vi "MoveToStrip.vi"(6 "Single Needle":bool, 8 "Error In":errorcluster, 9 "Strip No.":u16, 10 "Region":u16, 11 "ProbeStationControl in":refnum<class "ProbeStationControl.lvclass">) -> (0 "Error Out":errorcluster, 2 "Z [µm]":i32, 3 "ProbeStationControl out":refnum<class "ProbeStationControl.lvclass">)   [LabVIEW 2018]
doc: "Move to specified strip index and touch down probe."
uses:
  InstrControl/ProbeStationControl/ProbeStationControl.lvclass
  InstrControl/ProbeStationControl/TeslaVelox/TeslaVeloxProbeStation.lvclass
  ProbePlanParams.vi
panel:
  out "Is Valid?":bool
  out "Axis":enum16{"X", "Y", "Z", "Theta"}(ring)
  out "Coordinate IN":i32
  out "Coordinate system":enum16{"Cartesian", "X as index"}(ring)
  out "previous Z [µm]":i32
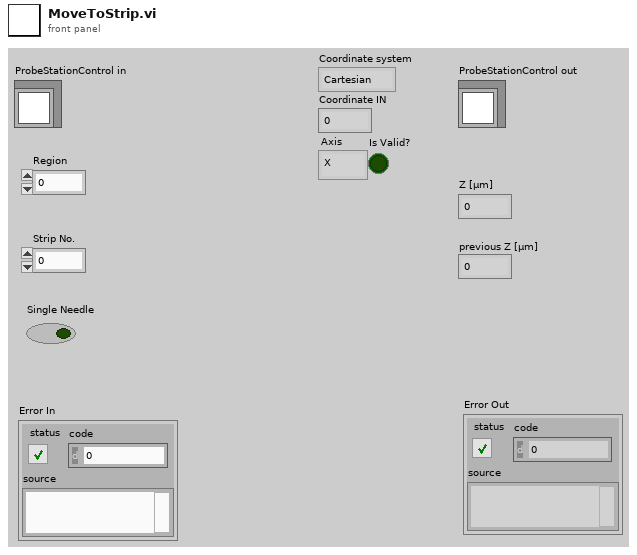
[diagram p1: front panel]
types:
  T1 = cluster{"Strip Number OUT":i32, "X0":i32, "Y0":i32, "X1":i32, "Y1":i32, "Xref":dbl, "Yref":dbl, "ProbePlan type":u32, "Inner pads offset":ext, "Outer pads offset":ext, "l_inner":ext, "l_outer":ext, "strip numbering":u16, "Device Orientation":ext, "Stagger offset":i32, "Yoffset":dbl, "Strip pitch":dbl, "Fiducail separation":dbl, "Radius":ext, "Relative strip angles":dbl, "Probeplan description":string, "ProbePlan array":cluster{"Region":string, "ProbePoints":cluster{"X":dbl, "Y":dbl, "Label":string, "CardViable?":bool}[]}[], "Test ProbePoints":cluster{"Regions Enabled":bool[], "From index":u32[], "To index":u32[]}}
  T2 = cluster{"Region":string, "ProbePoints":cluster{"X":dbl, "Y":dbl, "Label":string, "CardViable?":bool}[]}[]
  T3 = cluster{"Region":string, "ProbePoints":cluster{"X":dbl, "Y":dbl, "Label":string, "CardViable?":bool}[]}
  T4 = cluster{"X":dbl, "Y":dbl, "Label":string, "CardViable?":bool}[]
  T5 = cluster{"X":dbl, "Y":dbl, "Label":string, "CardViable?":bool}
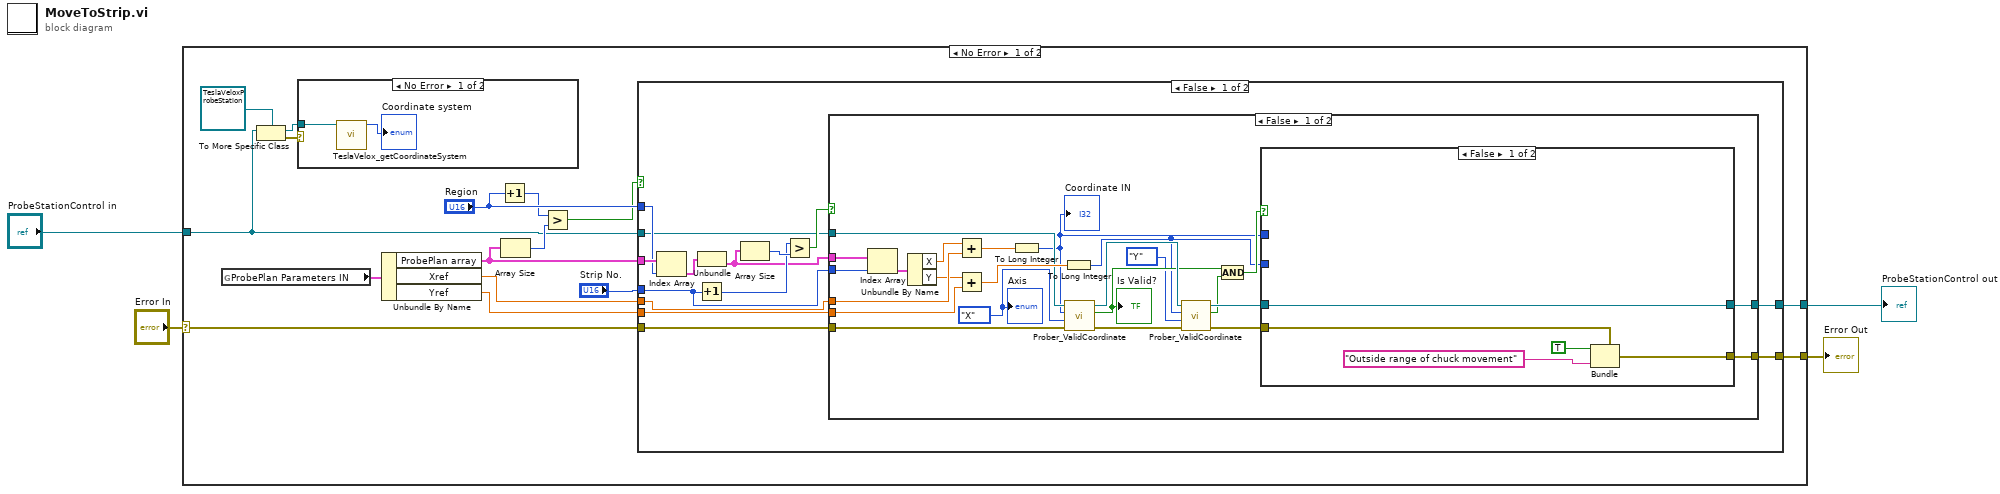
[diagram p0: block diagram]
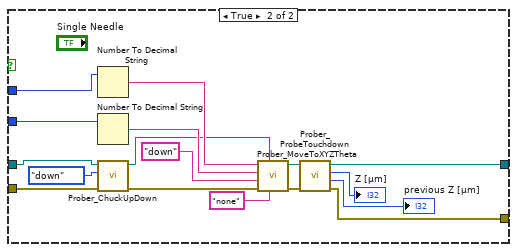
[diagram p3: hidden frame]
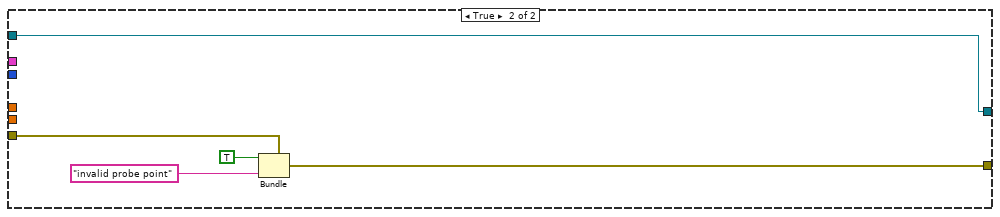
[diagram p4: hidden frame]
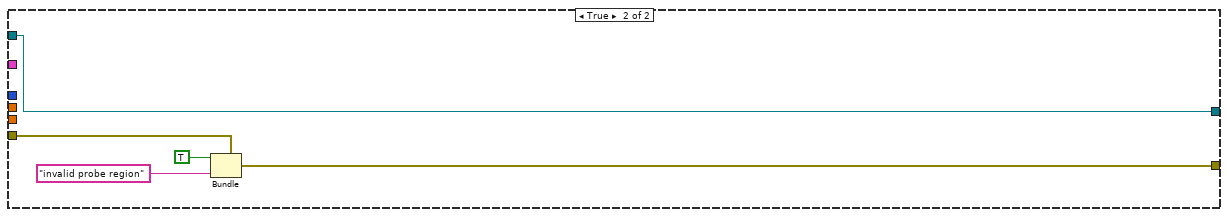
[diagram p5: hidden frame]
diagram:
  n1 = case shown="No Error" "Error In" {
    selector: "Error In" -> [w14 w93]
    tunnel: [w20 w93] -> w4
    tunnel: "ProbeStationControl in" -> [w8 w94]
    tunnel: [w9 w94] -> w1
    frame No Error {
      n2 = global read "ProbePlanParams.vi" "ProbePlan Parameters IN"() -> (w13:T1)
      n3 = To More Specific Class(target class=refnum<class "TeslaVeloxProbeStation.lvclass"> refnum ("TeslaVeloxProbeStation.lvclass"), reference=w8) -> (specific class reference=w7:refnum<class "TeslaVeloxProbeStation.lvclass">, error out=w5:errorcluster)  [unwired: 1 in]
      n4 = case shown="No Error" w5 {
        tunnel: w7 -> [w22 _]
        frame No Error {
          n5 = call "TeslaVelox_getCoordinateSystem.vi"("TeslaVeloxProbeStation.lvclass"=w22) -> ("Coordinate system"=→"Coordinate system":enum16{"Cartesian", "X as index"})  [unwired: 10 in]
        }
        frame Error {
        }
      }
      n6 = Unbundle By Name(w13) -> ("ProbePlan array"=w12:T2, "Xref"=w11:dbl, "Yref"=w10:dbl)
      n7 = Increment(x="Region") -> (x+1=w16:u16)
      n8 = Array Size(array=w12) -> (size(s)=w17:i32)
      n9 = Greater?(x=w16, y=w17) -> (0:w15:bool)
      n10 = case shown="False" w15 {
        tunnel: w14 -> [w31 w92]
        tunnel: [w30 w91] -> w20
        tunnel: "Region" -> [w34 _]
        tunnel: "Strip No." -> [w25 _]
        tunnel: w12 -> [w35 _]
        tunnel: w10 -> [w28 _]
        tunnel: w11 -> [w27 _]
        tunnel: [w24 w88] -> w9
        tunnel: w8 -> [w23 w88]
        frame False {
          n11 = Index Array(array=w35, index=w34) -> (element=w36:T3)
          n12 = Increment(x=w25) -> (x+1=w32:u16)
          n13 = Unbundle(w36) -> ("ProbePoints"=w26:T4)  [unwired: 1 out]
          n14 = Array Size(array=w26) -> (size(s)=w33:i32)
          n15 = Greater?(x=w32, y=w33) -> (0:w29:bool)
          n16 = case shown="False" w29 {
            tunnel: w31 -> [w48 w86]
            tunnel: [w53 w85] -> w30
            tunnel: w28 -> [w60 _]
            tunnel: w27 -> [w59 _]
            tunnel: w26 -> [w58 _]
            tunnel: w25 -> [w57 _]
            tunnel: [w50 w83] -> w24
            tunnel: w23 -> [w49 w83]
            frame False {
              w37 = enum16{"X", "Y", "Z", "Theta"}."X" ("Axis")
              n17 = Index Array(array=w58, index=w57) -> (element=w56:T5)
              n18 = Unbundle By Name(w56) -> ("X"=w55:dbl, "Y"=w54:dbl)
              n19 = Add(x=w55, y=w59) -> (x+y=w52:dbl)
              n20 = Add(x=w54, y=w60) -> (x+y=w51:dbl)
              n21 = To Long Integer(number=w52) -> (32bit integer=w38:i32)
              "Coordinate IN" <- w38
              n22 = To Long Integer(number=w51) -> (32bit integer=w40:i32)
              n23 = call-dynamic "Prober_ValidCoordinate.vi"("error in (no error)"=w48, "Axis"=w37, "Coordinate IN"=w38, "ProbeStationControl in"=w49) -> ("error out"=w47:errorcluster, "Is Valid?"=w42:bool, "ProbeStationControl out"=w45:refnum<class "ProbeStationControl.lvclass">)  [unwired: 5 in]
              "Is Valid?" <- w42
              n24 = call-dynamic "Prober_ValidCoordinate.vi"("error in (no error)"=w47, "Axis"=enum16{"X", "Y", "Z", "Theta"}."Y", "Coordinate IN"=w40, "ProbeStationControl in"=w45) -> ("error out"=w46:errorcluster, "Is Valid?"=w43:bool, "ProbeStationControl out"=w44:refnum<class "ProbeStationControl.lvclass">)  [unwired: 5 in]
              n25 = And(x=w42, y=w43) -> (x .and. y?=w41:bool)
              n26 = case shown="False" w41 {
                tunnel: w46 -> [w63 w66]
                tunnel: [w62 w77] -> w53
                tunnel: w38 -> [_ w82]
                tunnel: w40 -> [_ w81]
                tunnel: [w61 w76] -> w50
                tunnel: w44 -> [w61 w67]
                frame False {
                  n27 = Bundle(cluster=w63, "status"=TRUE, "source"="Outside range of chuck movement") -> (w62:errorcluster)  [unwired: 1 in]
                }
                frame True {
                  n28 = Number To Decimal String(number=w82) -> (decimal integer string=w80:string)  [unwired: 1 in]
                  n29 = Number To Decimal String(number=w81) -> (decimal integer string=w79:string)  [unwired: 1 in]
                  n30 = call-dynamic "Prober_ChuckUpDown.vi"("error in (no error)"=w66, "Direction"=enum16{"up", "down"}."down", "ProbeStationControl in"=w67) -> ("error out"=w71:errorcluster, "ProbeStationControl out"=w72:refnum<class "ProbeStationControl.lvclass">)  [unwired: 6 in, 1 out]
                  n31 = call-dynamic "Prober_MoveToXYZTheta.vi"("Theta location [mdeg]"="none", "ProbeStationControl in"=w72, "error in (no error)"=w71, "Z location [µm]"="down", "Y location [µm]"=w79, "X location [µm]"=w80) -> ("error out"=w78:errorcluster, "ProbeStationControl out"=w75:refnum<class "ProbeStationControl.lvclass">)  [unwired: 3 in, 1 out]
                  n32 = call-dynamic "Prober_ProbeTouchdown.vi"("error in (no error)"=w78, "ProbeStationControl in"=w75) -> ("error out"=w77:errorcluster, "previous Z [µm]"=→"previous Z [µm]":i32, "Z [µm]"=→"Z [µm]":i32, "ProbeStationControl out"=w76:refnum<class "ProbeStationControl.lvclass">)  [unwired: 6 in]
                }
              }
              "Axis" <- w37
            }
            frame True {
              n33 = Bundle(cluster=w86, "status"=TRUE, "source"="invalid probe point") -> (w85:errorcluster)  [unwired: 1 in]
            }
          }
        }
        frame True {
          n34 = Bundle(cluster=w92, "status"=TRUE, "source"="invalid probe region") -> (w91:errorcluster)  [unwired: 1 in]
        }
      }
    }
    frame Error {
    }
  }
  "Error Out" <- w4
  "ProbeStationControl out" <- w1
